vi "User_Current_Read.vi"(8 "error in (no error)":errorcluster caption="错误输入（无错误）", 11 "Name":string) -> (0 "error out":errorcluster caption="错误输出", 3 "User_Info":T1 {"User_Right" items=["管理员", "操作员"]})   [LabVIEW 2020]
uses:
  User_Manage/User_Databse/User_Info.ctl
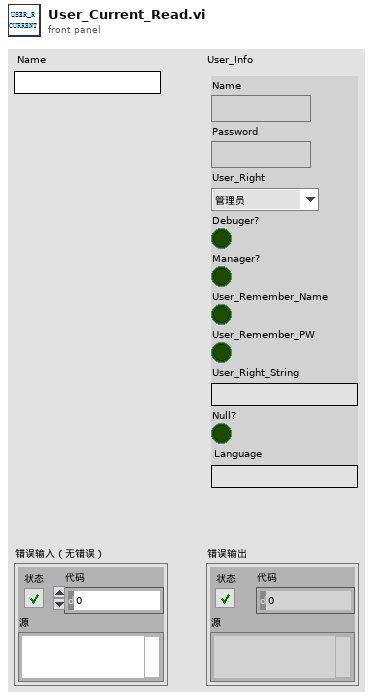
[diagram p1: front panel]
types:
  T1 = typedef "User_Info.ctl" = cluster{"Name":string, "Password":string, "User_Right":u16, "Debuger?":bool, "Manager?":bool, "User_Remember_Name":bool, "User_Remember_PW":bool, "User_Right_String":string, "Null?":bool, "Language":string}
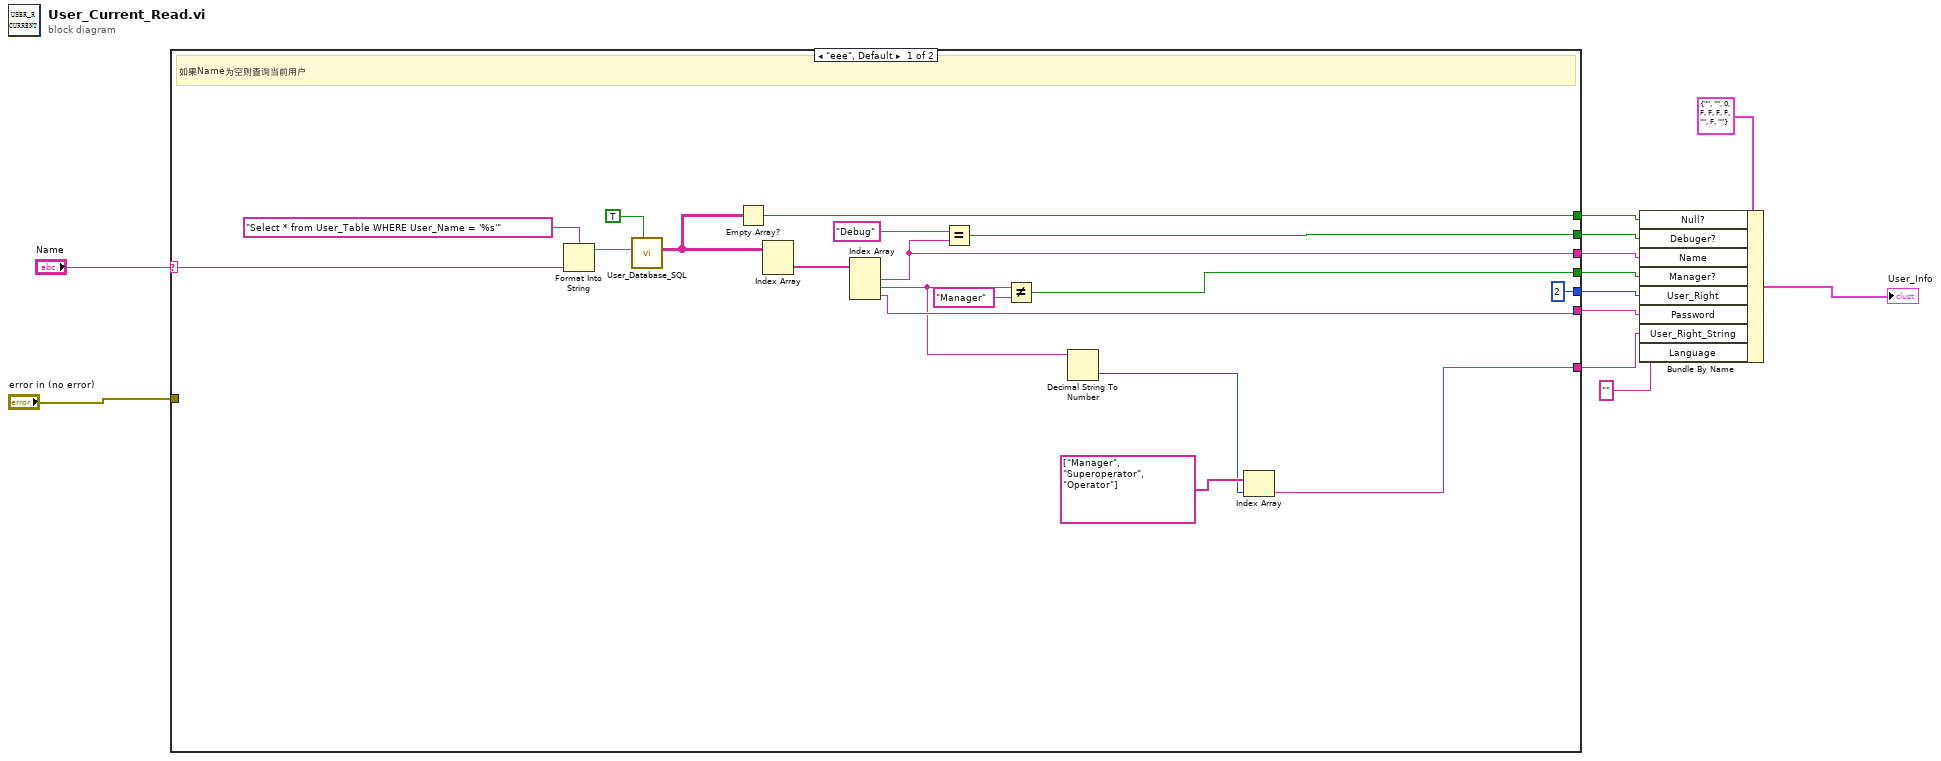
[diagram p0: block diagram]
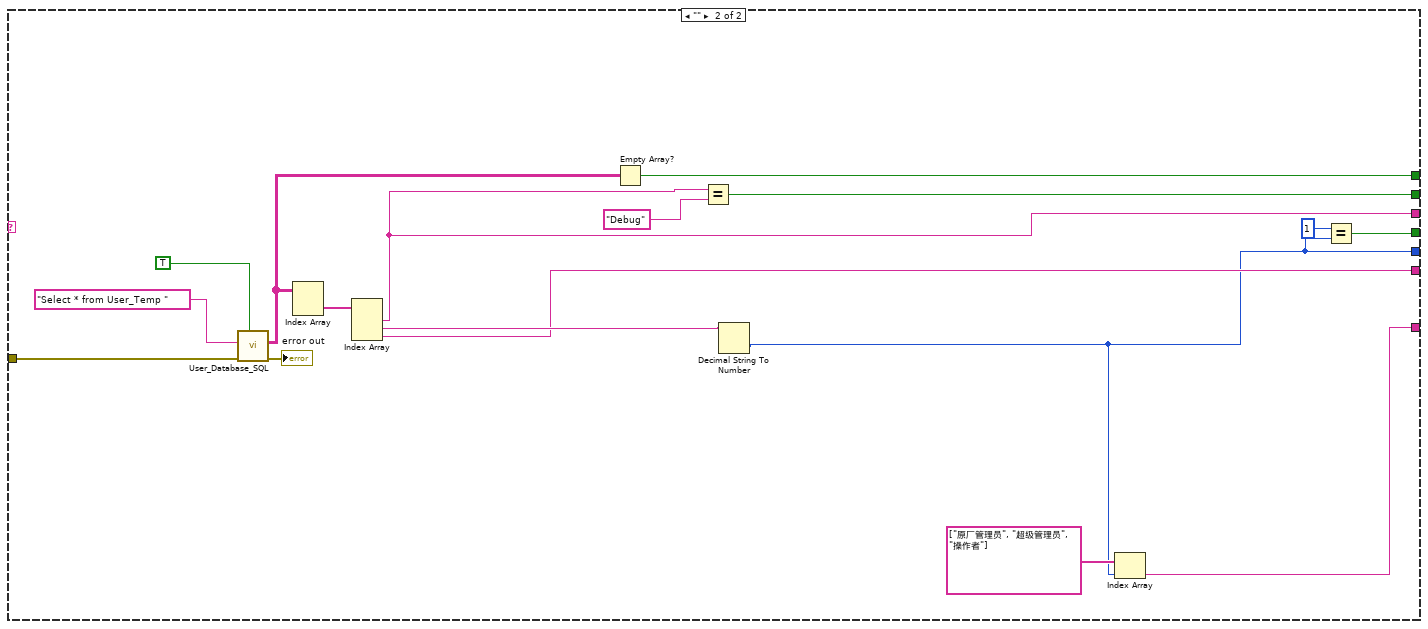
[diagram p2: hidden frame]
diagram:
  n1 = case shown="\"eee\", Default" "Name" {
    selector: "Name" -> [w27 _]
    tunnel: "error in (no error)" -> [_ w43]
    tunnel: [w24 w39] -> w11
    tunnel: [w23 w35] -> w10
    tunnel: [w20 w31] -> w9
    tunnel: [w21 w34] -> w8
    tunnel: [2 w33] -> w5
    tunnel: [w14 w36] -> w4
    tunnel: [w18 w40] -> w2
    frame "eee", Default {
      # "如果Name为空则查询当前用户"
      n2 = Format Into String(format string="Select * from User_Table WHERE User_Name = '%s'" ("SQL query"), w27) -> (resulting string=w30:string)  [unwired: 2 in, 1 out]
      n3 = call "User_Database_SQL.vi"("Get Record"=TRUE, "SQL query"=w30) -> ("Record"=w19:string[][])  [unwired: 7 in, 2 out]
      n4 = Empty Array?(array=w19) -> (empty?=w18:bool)
      n5 = Index Array(array=w19) -> (element=w26:string[])  [unwired: 2 in]
      n6 = Index Array(array=w26) -> (element #1=w23:string, element #2=w17:string, element #3=w21:string)  [unwired: 3 in]
      n7 = Equal?(x="Debug", y=w23) -> (x = y?=w24:bool)
      n8 = Not Equal?(x=w17, y="Manager") -> (x != y?=w20:bool)
      n9 = Decimal String To Number(string=w17) -> (number=w15:i32)  [unwired: 2 in, 1 out]
      n10 = Index Array(array=string[] ["Manager", "Superoperator", "Operator"] ("字符串数组"), index=w15) -> (element=w14:string)
    }
    frame "" {
      n11 = call "User_Database_SQL.vi"("Get Record"=TRUE, "error in (no error)"=w43, "SQL query"="Select * from User_Temp ") -> ("error out"=→"error out":errorcluster, "Record"=w41:string[][])  [unwired: 6 in, 1 out]
      n12 = Index Array(array=w41) -> (element=w45:string[])  [unwired: 2 in]
      n13 = Index Array(array=w45) -> (element #1=w35:string, element #2=w38:string, element #3=w34:string)  [unwired: 3 in]
      n14 = Empty Array?(array=w41) -> (empty?=w40:bool)
      n15 = Equal?(x=w35, y="Debug") -> (x = y?=w39:bool)
      n16 = Decimal String To Number(string=w38) -> (number=w33:i32)  [unwired: 2 in, 1 out]
      n17 = Index Array(array=string[] ["原厂管理员", "超级管理员", "操作者"] ("字符串数组"), index=w33) -> (element=w36:string)
      n18 = Equal?(x=1, y=w33) -> (x = y?=w31:bool)
    }
  }
  n19 = Bundle By Name(cluster=T1 {"Name"="", "Password"="", "User_Right"=0, "Debuger?"=FALSE, "Manager?"=FALSE, "User_Remember_Name"=FALSE, "User_Remember_PW"=FALSE, "User_Right_String"="", "Null?"=FALSE, "Language"=""} ("簇"), "Null?"=w2, "Debuger?"=w11, "Name"=w10, "Manager?"=w9, "User_Right"=w5, "Password"=w8, "User_Right_String"=w4, "Language"="") -> (→"User_Info":T1)
